vi "New Logger.vi"(4 "dialog on failure? (T)":bool=TRUE, 5 "minimum log level (Info)":T1=enum."Info", 6 "enabled? (T)":bool=TRUE, 7 "name (\"Default\")":string="Default", 8 "error in (no error)":errorcluster, 9 "log handler (file handler)":refnum<class "Formatting Handler.lvclass">, 10 "log filter (none)":refnum<class "Filter.lvclass">, 11 "logger scope (all)":refnum<class "Scope.lvclass">) -> (0 "error out":errorcluster, 3 "logger":refnum<class "Logger.lvclass">)   [LabVIEW 2018, in "GLog.lvlib" / "Logger.lvclass"]
uses:
  Logger.lvclass
  extension/scope_interface/Scope.lvclass
  extension/formatting_handler_interface/Formatting Handler.lvclass
  extension/filter_interface/Filter.lvclass
  Log Levels.ctl
  Logger.lvclass/Logger.ctl
  configuration/handlers/file_handler/File Handler.lvclass
  C:/Users/Colin/Documents/software_projects/labview/glog/src/api/extension/formatting_handler_interface/Formatting Handler.lvclass
  GLog.lvlib
panel:
  # "Connector Pane"
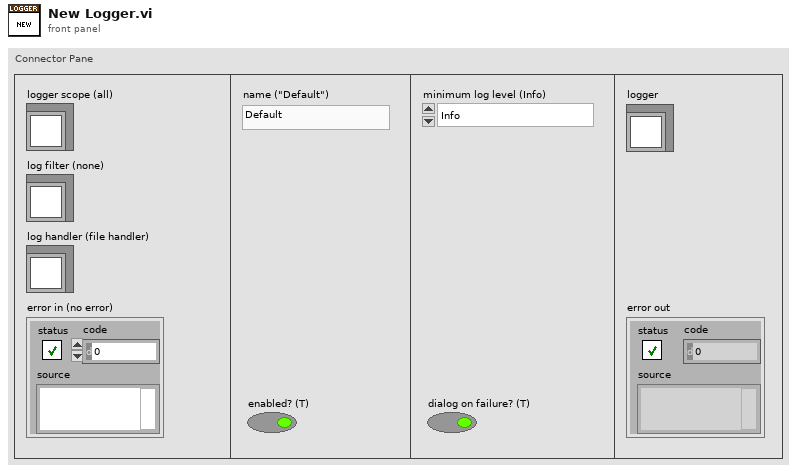
[diagram p1: front panel]
types:
  T1 = typedef "GLog.lvlib/Log Levels.ctl" = enum16{"Trace", "Debug", "Info", "Warning", "Error", "Critical"}
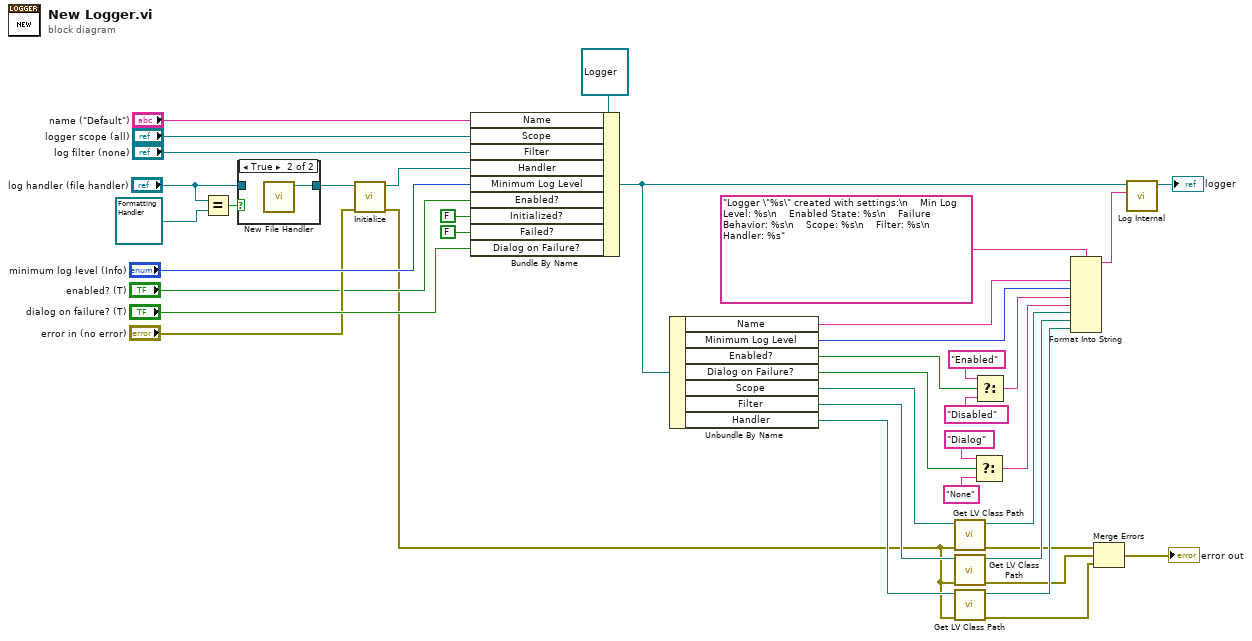
[diagram p0: block diagram]
diagram:
  n1 = Equal?(x="log handler (file handler)", y=refnum<class "Formatting Handler.lvclass"> refnum ("log handler (file handler)")) -> (x = y?=w27:bool)
  n2 = case shown="True" w27 {
    tunnel: [w41 w42] -> w37
    tunnel: "log handler (file handler)" -> [w41 _]
    frame False {
    }
    frame True {
      n3 = call "New File Handler.vi"() -> ("file handler"=w42:refnum<class "File Handler.lvclass">)  [unwired: 11 in]
    }
  }
  n4 = call-dynamic "Initialize.vi"("error in (no error)"="error in (no error)", "handler in"=w37) -> ("error out"=w5:errorcluster, "handler out"=w35:refnum<class "Formatting Handler.lvclass">)  [unwired: 8 in]
  n5 = Bundle By Name(cluster=refnum<class "Logger.lvclass"> refnum ("logger"), "Name"="name (\"Default\")", "Scope"="logger scope (all)", "Filter"="log filter (none)", "Handler"=w35, "Minimum Log Level"="minimum log level (Info)", "Enabled?"="enabled? (T)", "Initialized?"=FALSE ("Active?"), "Failed?"=FALSE, "Dialog on Failure?"="dialog on failure? (T)") -> (w25:refnum<class "Logger.lvclass">)
  n6 = Unbundle By Name(w25) -> ("Name"=w22:string, "Minimum Log Level"=w21:T1, "Enabled?"=w20:bool, "Dialog on Failure?"=w15:bool, "Scope"=w11:refnum<class "Scope.lvclass">, "Filter"=w10:refnum<class "Filter.lvclass">, "Handler"=w9:refnum<class "Formatting Handler.lvclass">)
  n7 = call <vilib>:"Get LV Class Path.vi"("error in (no error)"=w5, "object"=w11) -> ("error out"=w4:errorcluster, "class path"=w8:path)  [unwired: 8 in]
  n8 = call <vilib>:"Get LV Class Path.vi"("error in (no error)"=w5, "object"=w10) -> ("error out"=w3:errorcluster, "class path"=w7:path)  [unwired: 8 in]
  n9 = call <vilib>:"Get LV Class Path.vi"("error in (no error)"=w5, "object"=w9) -> ("error out"=w2:errorcluster, "class path"=w6:path)  [unwired: 8 in]
  n10 = Select(t="Dialog", s=w15, f="None") -> (s? t:f=w13:string)
  n11 = Select(t="Enabled", s=w20, f="Disabled") -> (s? t:f=w17:string)
  n12 = Format Into String(format string="Logger \"%s\" created with settings:\n    Min Log Level: %s\n    Enabled State: %s\n    Failure Behavior: %s\n    Scope: %s\n    Filter: %s\n    Handler: %s" ("message"), w22, w21, w17, w13, w8, w7, w6) -> (resulting string=w24:string)  [unwired: 2 in, 1 out]
  n13 = Merge Errors(w4, w3, w2) -> (→"error out":errorcluster)
  n14 = call "Log Internal.vi"("message"=w24, "logger in"=w25) -> ("logger out"=→"logger":refnum<class "Logger.lvclass">)  [unwired: 9 in]
